vi "CalcBlobLocation.vi"(5 "TargetCameraAngleOffset (deg)":cluster{"X":dbl, "Y":dbl}={"X"=66.5, "Y"=0.0}, 6 "Camera Distance":dbl=268.0, 7 "RefCameraAngleOffset (deg)":cluster{"X":dbl, "Y":dbl}={"X"=66.5, "Y"=0.0}, 8 "Camera View Angles (deg)":cluster{"X":dbl, "Y":dbl}={"X"=47.0, "Y"=32.5}, 9 "ImageSize  (px)":cluster{"X":i32, "Y":i32}, 10 "TargetBlob (px)":cluster{"X":i32, "Y":i32}, 11 "RefBlob (px)":cluster{"X":i32, "Y":i32}) -> (0 "Side b":dbl, 1 "Side a":dbl, 2 "Distance":dbl, 3 "Angle C":dbl, 4 "Area":dbl)   [LabVIEW 2011]
uses:
  <vilib>/Analysis/coordinate.llb/Angle Units.ctl
  <vilib>/Analysis/coordinate.llb/Supplementary Angle (scalar).vi
  <vilib>/Analysis/coordinate.llb/Wrap Angle (scalar).vi
  <vilib>/Analysis/coordinate.llb/Set Angle Unit.vi
  <vilib>/Analysis/NI_AAL_Angle.lvlib
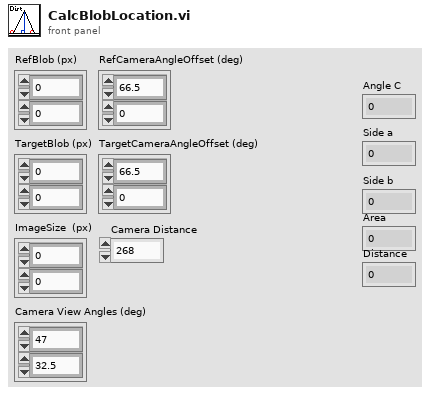
[diagram p1: front panel]
types:
  T1 = typedef "NI_AAL_Angle.lvlib/Angle Units.ctl" = i32
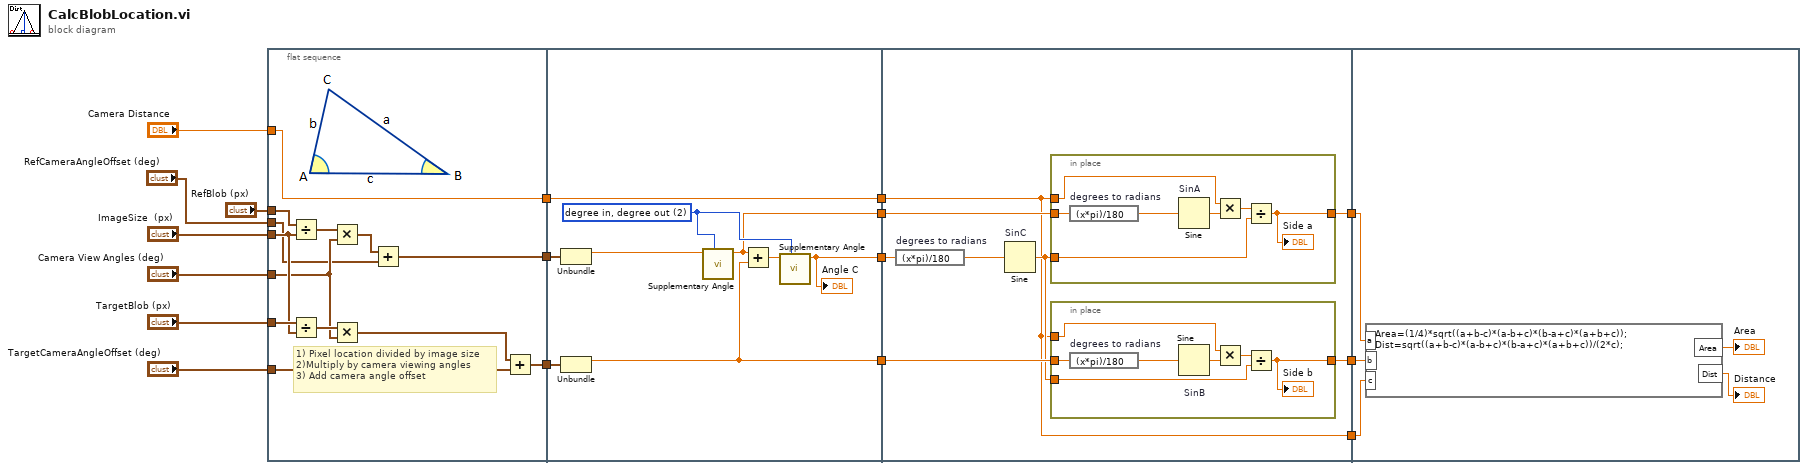
[diagram p0: block diagram]
diagram:
  n1 = flat-sequence {
    tunnel: "ImageSize  (px)" -> [w28]
    tunnel: "RefBlob (px)" -> [w30]
    tunnel: "TargetBlob (px)" -> [w29]
    tunnel: "Camera View Angles (deg)" -> [w26]
    tunnel: "RefCameraAngleOffset (deg)" -> [w23]
    tunnel: "TargetCameraAngleOffset (deg)" -> [w21]
    tunnel: [w20] -> w11
    tunnel: [w19] -> w10
    tunnel: [w18] -> w9
    tunnel: "Camera Distance" -> [w18]
    tunnel: w11 -> [w38]
    tunnel: w10 -> [w39]
    tunnel: w9 -> [w33]
    tunnel: [w34] -> w7
    tunnel: [w32] -> w6
    tunnel: [w31] -> w5
    tunnel: [w33] -> w4
    tunnel: w7 -> [w47]
    tunnel: w6 -> [w46]
    tunnel: w5 -> [w44]
    tunnel: w4 -> [w40]
    tunnel: [w42] -> w3
    tunnel: [w41] -> w2
    tunnel: [w40] -> w1
    tunnel: w3 -> [w66]
    tunnel: w2 -> [w65]
    tunnel: w1 -> [w64]
    frame #0 {
      # "1) Pixel location divided by image size\n2)Multiply by camera viewing angles\n3) Add camera angle offset"
      n2 = Divide(x=w30, y=w28) -> (x/y=w25:cluster{"X":dbl, "Y":dbl})
      n3 = Divide(x=w29, y=w28) -> (x/y=w27:cluster{"X":dbl, "Y":dbl})
      n4 = Multiply(x=w25, y=w26) -> (x*y=w24:cluster{"X":dbl, "Y":dbl})
      n5 = Multiply(x=w27, y=w26) -> (x*y=w22:cluster{"X":dbl, "Y":dbl})
      n6 = Add(x=w24, y=w23) -> (x+y=w19:cluster{"X":dbl, "Y":dbl})
      n7 = Add(x=w22, y=w21) -> (x+y=w20:cluster{"X":dbl, "Y":dbl})
    }
    frame #1 {
      w36 = T1 2 items=["radian in, radian out", "radian in, degree out", "degree in, degree out", "degree in, radian out"] ("angle units")
      n8 = Unbundle(w39) -> ("X"=w35:dbl)  [unwired: 1 out]
      n9 = Unbundle(w38) -> ("X"=w32:dbl)  [unwired: 1 out]
      n10 = call-poly <vilib>:"Supplementary Angle.vi"("angle units"=w36, "angle"=w35) -> ("supplementary angle"=w34:dbl)  [unwired: 8 in, 1 out]
      n11 = Add(x=w34, y=w32) -> (x+y=w37:dbl)
      n12 = call-poly <vilib>:"Supplementary Angle.vi"("angle units"=w36, "angle"=w37) -> ("supplementary angle"=w31:dbl)  [unwired: 8 in, 1 out]
      "Angle C" <- w31
    }
    frame #2 {
      n13 = expression code="(x*pi)/180" "degrees to radians"(w44) -> (w43:dbl)
      n14 = Sine "SinC"(x=w43) -> (sin(x)=w45:dbl)
      n15 = in-place {
        in-place-border: w47 -> [w54]
        in-place-border: w40 -> [w51]
        in-place-border: w45 -> [w50]
        in-place-border: [w48] -> w42
        n16 = expression code="(x*pi)/180" "degrees to radians"(w54) -> (w49:dbl)
        n17 = Sine "SinA"(x=w49) -> (sin(x)=w53:dbl)
        n18 = Multiply(x=w51, y=w53) -> (x*y=w52:dbl)
        n19 = Divide(x=w52, y=w50) -> (x/y=w48:dbl)
        "Side a" <- w48
      }
      n20 = in-place {
        in-place-border: w46 -> [w57]
        in-place-border: w40 -> [w60]
        in-place-border: w45 -> [w58]
        in-place-border: [w55] -> w41
        n21 = expression code="(x*pi)/180" "degrees to radians"(w57) -> (w56:dbl)
        n22 = Sine "SinB"(x=w56) -> (sin(x)=w59:dbl)
        n23 = Multiply(x=w60, y=w59) -> (x*y=w61:dbl)
        n24 = Divide(x=w61, y=w58) -> (x/y=w55:dbl)
        "Side b" <- w55
      }
    }
    frame #3 {
      n25 = formula code="Area=(1/4)*sqrt((a+b-c)*(a-b+c)*(b-a+c)*(a+b+c));\nDist=sqrt((a+b-c)*(a-b+c)*(b-a+c)*(a+b+c))/(2*c);"("a"=w66, "b"=w65, "c"=w64) -> ("Area"=→"Area":dbl, "Dist"=→"Distance":dbl)
    }
  }
